vi "open subVI by relative path.vi"(8 "error in":errorcluster, 10 "relative path":string, 11 "project in":refnum<vi>) -> (0 "error out":errorcluster, 2 "vi reference":refnum<vi>, 3 "project out":refnum<vi>)   [LabVIEW 2013, in "DecideModuleFeatures.lvclass"]
uses:
  DecideModuleFeatures.lvclass
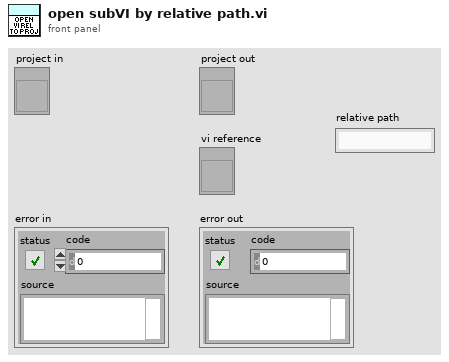
[diagram p1: front panel]
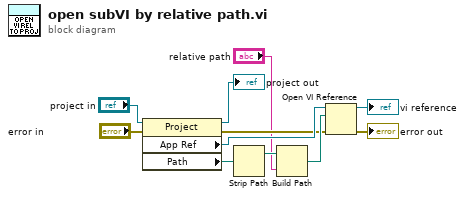
[diagram p0: block diagram]
diagram:
  n1 = property class="Project"(reference="project in", error in="error in") -> (reference out=→"project out":refnum<vi>, error out=w3:errorcluster, "App Ref"=w4:refnum<vi>, "Path"=w2:path)
  n2 = Strip Path(path=w2) -> (stripped path=w11:path)  [unwired: 1 out]
  n3 = Build Path(base path=w11, name or relative path="relative path") -> (appended path=w5:path)
  n4 = Open VI Reference(application reference (local)=w4, vi path=w5, error in (no error)=w3) -> (vi reference=→"vi reference":refnum<vi>, error out=→"error out":errorcluster)  [unwired: 3 in]
